vi "Frame Configuration Page.vi"(8 "error in (no error)":errorcluster, 11 "Node Ptr":T2 format="%.0x") -> (0 "error out":errorcluster)   [LabVIEW 2021, in "LIN Frame Protection Addon System Explorer.lvlib"]
uses:
  LIN Frame Protection Addon System Explorer.lvlib
  <vilib>/NI VeriStand/Custom Device API/Custom Device Item Ref.ctl
  Shared/Types/Protection Type.ctl
  <vilib>/NI VeriStand/Custom Device API/Custom Device API.lvlib
  Shared/LIN Frame Protection Addon Shared.lvlib
panel:
  out "Delays (s)":string
  in  "Protection Type":T1
  out "Frame ID":u32 format="%.0x"
  in  "Max Count":dbl=4.0
  out "Rolling Counter Channel":string
  out "CRC Channel":string
  in  "SHDocVw.IWebBrowser":refnum<k7>(container)
  in  "Value":dbl
  in  "Monitored Channels":i32(listbox)
  in  "Header":cluster{"Section Name":string}={"Section Name"="Custom Device Item Settings"}
  in  "Description":string
  in  "Name":string
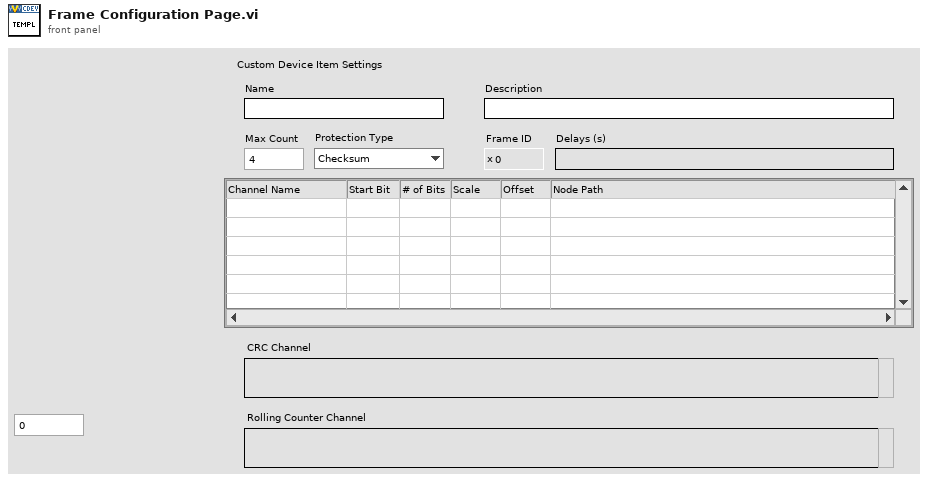
[diagram p1: front panel]
types:
  T1 = typedef "LIN Frame Protection Addon Shared.lvlib/Protection Type.ctl" = enum16{"Checksum", "CRC", "None (Counter Only)"}
  T2 = typedef "Custom Device API.lvlib/Custom Device Item Ref.ctl" = u64
  T3 = typedef "Custom Device API.lvlib/Custom Device Item Info.ctl" = cluster{"Name":string, "Is Channel":bool, "GUID":string, "Is Waveform":bool}
  T4 = typedef "LIN Frame Protection Addon Shared.lvlib/FrameConfiguration.ctl" = cluster{"Input Channels":T5[], "Schedule_SumOfDelays":cluster{"Index":i32, "Delays":dbl[]}, "Rolling Counter Count":dbl, "PCL Count":u64, "Max Count":dbl, "Frame ID":u32, "Rolling Counter":T5, "CRC":T5, "Frame Name":string, "Cluster":string, "Database":string, "Protection Type":T1}
  T5 = typedef "LIN Frame Protection Addon Shared.lvlib/InputChannelConfiguration.ctl" = cluster{"Start Bit":i32, "Name":string, "Node Path":string, "Number of bits":i32, "Scale":dbl, "Offset":dbl, "Data Type":u32}
  T6 = typedef "Custom Device API.lvlib/Custom Device Commands.ctl" = enum16{"Default", "Item renamed", "Shutdown", "Dynamic button pressed"}
  T7 = typedef "LVPoint32TypeDef.ctl" = cluster{"Horizontal":i32, "Vertical":i32}
  T8 = typedef "LVRowAndColumnTypeDef.ctl" = cluster{"Row":i32, "Column":i32}
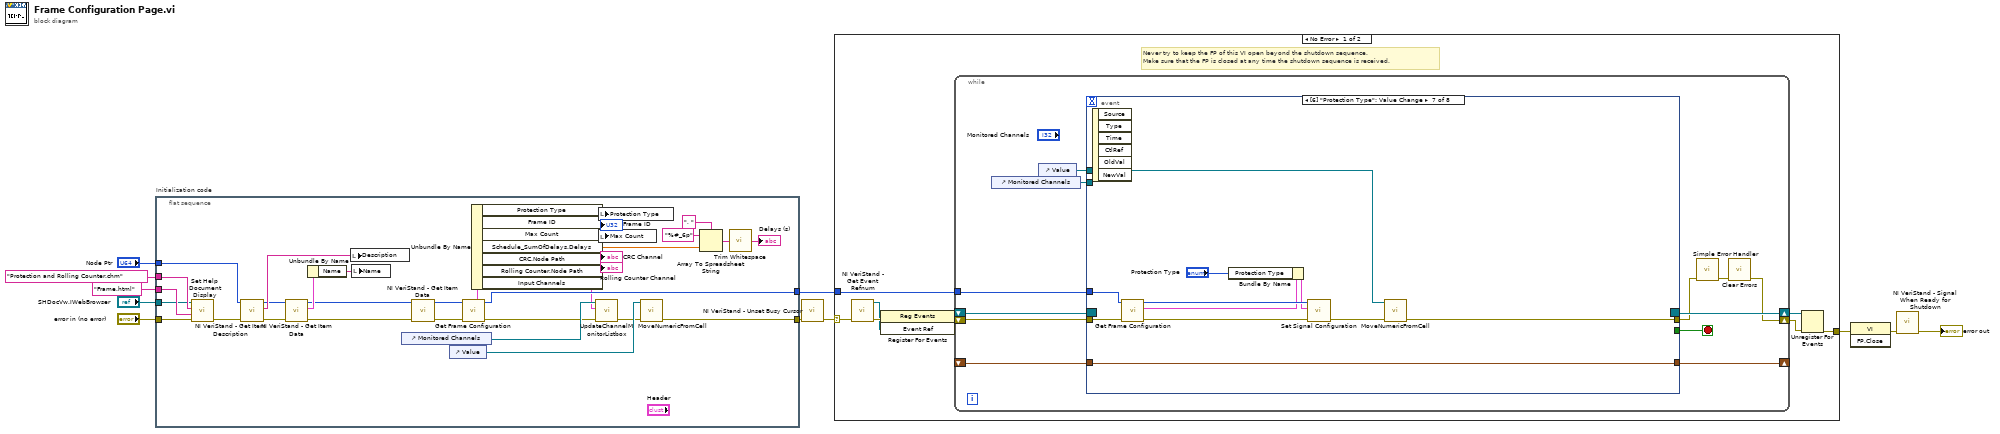
[diagram p0: block diagram]
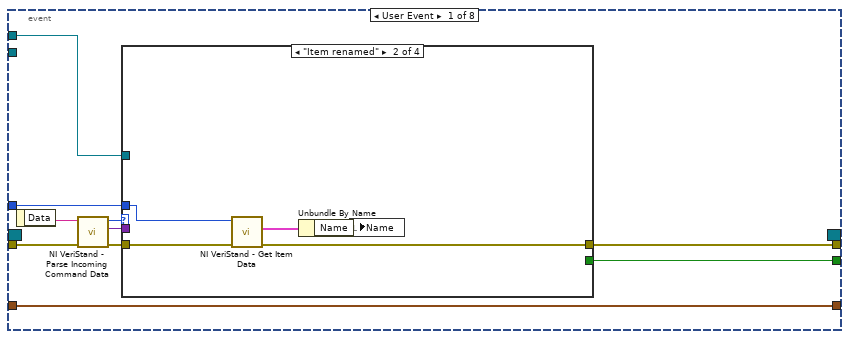
[diagram p2: hidden frame]
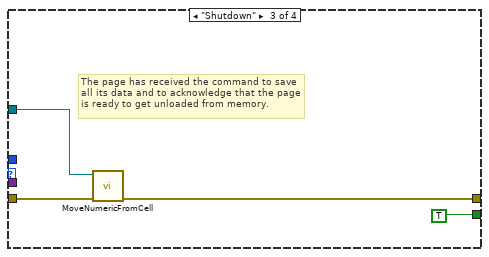
[diagram p4: hidden frame]
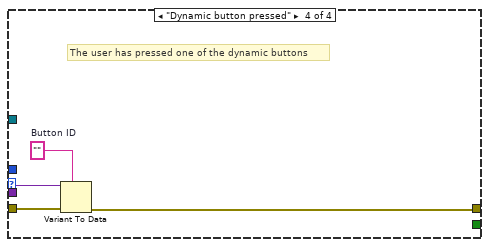
[diagram p5: hidden frame]
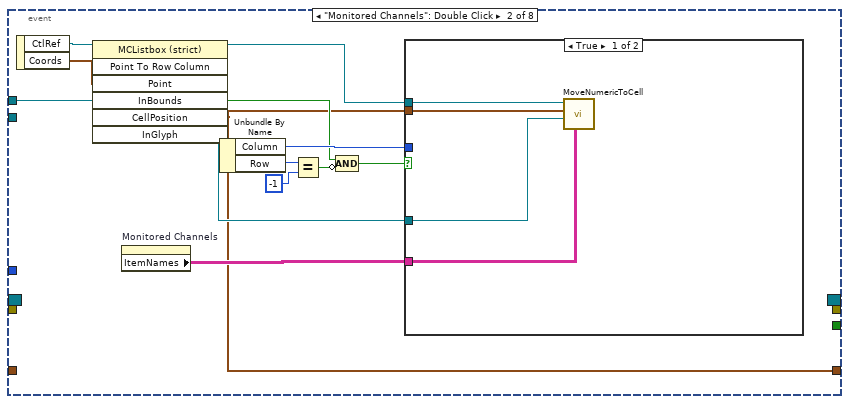
[diagram p6: hidden frame]
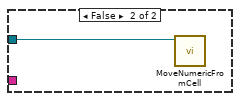
[diagram p7: hidden frame]
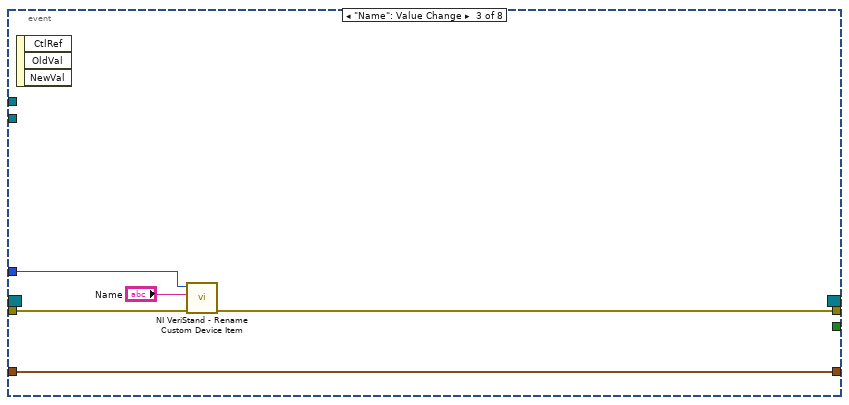
[diagram p8: hidden frame]
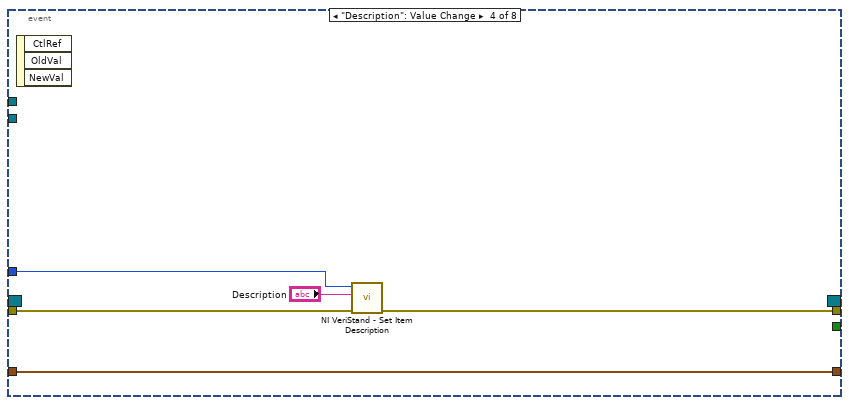
[diagram p9: hidden frame]
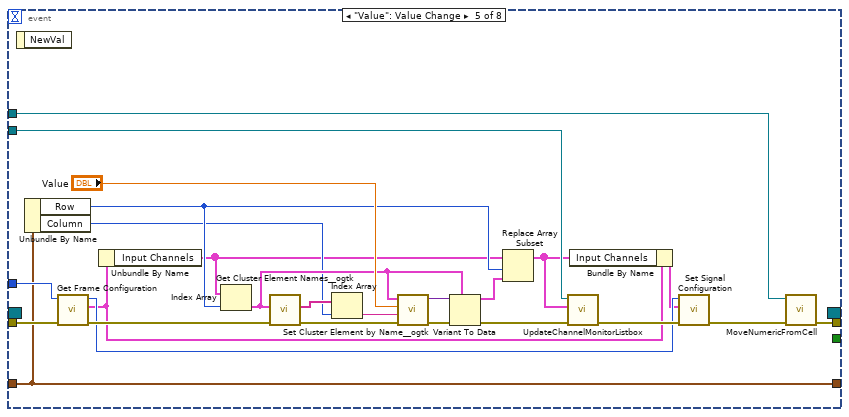
[diagram p10: hidden frame]
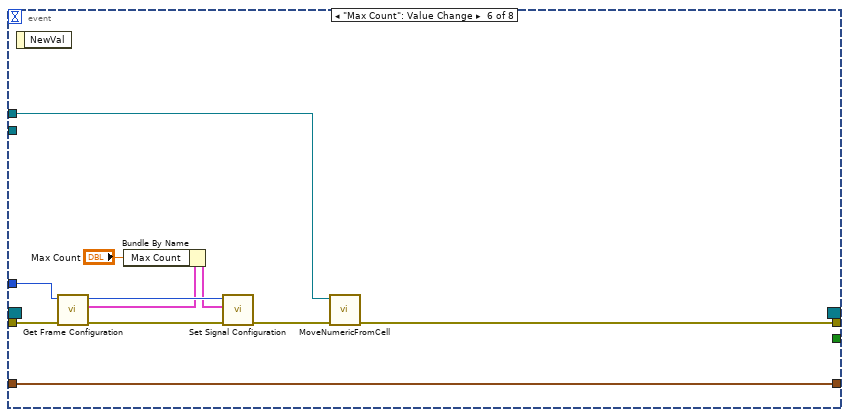
[diagram p11: hidden frame]
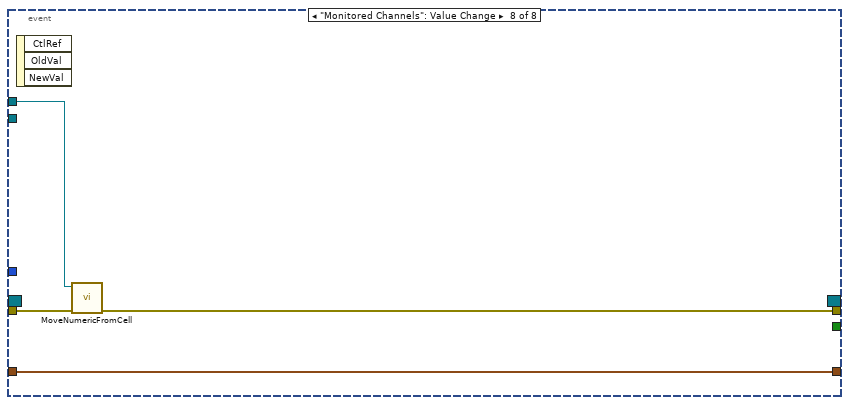
[diagram p12: hidden frame]
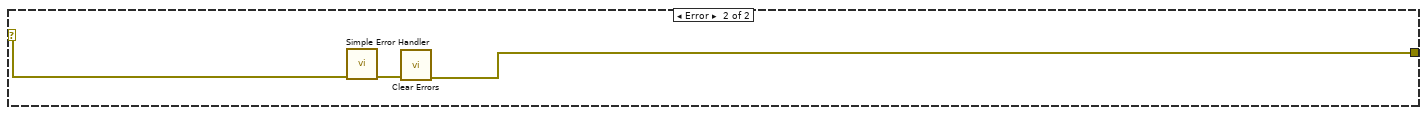
[diagram p13: hidden frame]
diagram:
  n1 = flat-sequence "Initialization code" {
    tunnel: "error in (no error)" -> [w35]
    tunnel: "Node Ptr" -> [w23]
    tunnel: [w32] -> w9
    tunnel: [w40] -> w7
    tunnel: "Protection and Rolling Counter.chm" ("Main CHM File") -> [w44]
    tunnel: "Frame.html" ("HTML File") -> [w43]
    tunnel: "SHDocVw.IWebBrowser" -> [w42]
    frame #0 {
      n2 = call "Set Help Document Display.vi"("error in (no error)"=w35, "HTML File"=w43, "Main CHM File"=w44, "SHDocVw.IWebBrowser2"=w42) -> ("error out"=w25:errorcluster)  [unwired: 7 in]
      n3 = call <vilib>:"NI VeriStand - Get Item Description.vi"("error in (no error)"=w25, "Item Ref in"=w23) -> ("error out"=w28:errorcluster, "Description"=w27:string, "Item Ref out"=w26:T2)  [unwired: 7 out]
      n4 = call <vilib>:"NI VeriStand - Get Item Data.vi"("error in (no error)"=w28, "Item Ref in"=w26) -> ("error out"=w24:errorcluster, "Item Info"=w29:T3, "Item Ref out"=w22:T2)  [unwired: 7 out]
      n5 = Unbundle By Name(w29) -> ("Name"=w30:string)
      n6 = local write "Description"(w27) -> ()
      n7 = local write "Name"(w30) -> ()
      n8 = control-ref of="Monitored Channels"() -> (w37:refnum<vi>)
      n9 = call <vilib>:"NI VeriStand - Get Item Data.vi"("error in (no error)"=w24, "Item Ref in"=w22) -> ("error out"=w39:errorcluster, "Item Ref out"=w41:T2)  [unwired: 8 out]
      n10 = control-ref of="Value"() -> (w34:refnum<vi>)
      n11 = call "Get Frame Configuration.vi"("error in"=w39, "Parent Ref"=w41) -> ("error out"=w36:errorcluster, "Selected Channels"=w38:T4, "Parent Ref Out"=w40:T2)  [unwired: 7 in]
      n12 = Unbundle By Name(w38) -> ("Protection Type"=w17:T1, "Frame ID"=→"Frame ID":u32, "Max Count"=w19:dbl, "Schedule_SumOfDelays.Delays"=w16:dbl[], "CRC.Node Path"=→"CRC Channel":string, "Rolling Counter.Node Path"=→"Rolling Counter Channel":string, "Input Channels"=w31:T5[])
      n13 = call "UpdateChannelMonitorListbox.vi"("error in (no error)"=w36, "Monitored Channels"=w31, "Listbox"=w37) -> ("error out"=w33:errorcluster)  [unwired: 8 in]
      n14 = local write "Protection Type"(w17) -> ()
      n15 = local write "Max Count"(w19) -> ()
      n16 = call "MoveNumericFromCell.vi"("error in (no error)"=w33, "Digital in"=w34) -> ("error out"=w32:errorcluster)  [unwired: 9 in]
      n17 = Array To Spreadsheet String(delimiter (Tab)=", ", array=w16, 3:"%#_6p" ("format string")) -> (spreadsheet string=w15:string)
      n18 = call <vilib>:"Trim Whitespace.vi"("string"=w15) -> ("trimmed string"=→"Delays (s)":string)  [unwired: 1 in]
    }
  }
  n19 = call <vilib>:"NI VeriStand - Unset Busy Cursor.vi"("error in (no error)"=w9) -> ("error out"=w8:errorcluster)  [unwired: 10 out]
  n20 = case shown="No Error" w8 {
    selector: w8 -> [w45 w170]
    tunnel: [w50 w168] -> w11
    tunnel: w7 -> [w46 _]
    frame No Error {
      # "Never try to keep the FP of this VI open beyond the shutdown sequence.\nMake sure that the FP is closed at any time the shutdown sequence is received."
      n21 = call <vilib>:"NI VeriStand - Get Event Refnum.vi"("error in (no error)"=w45) -> ("error out"=w53:errorcluster, "Event Ref"=w49:refnum<user-event>)  [unwired: 9 out]
      n22 = register-events(error in=w53, w49) -> (reference out=w47:refnum<event-registration>, error out=w48:errorcluster)  [unwired: 1 in]
      n23 = while {
        tunnel: w46 -> [w61]
        shift-right: [w58] -> w51
        shift-left: w48 -> [w64]
        shift-right: [w65] -> w52
        shift-left: w47 -> [w63]
        shift-right: [w56] -> _
        shift-left: _ -> [w55]
        stop <- w62 stop-if-true
        n24 = control-ref of="Monitored Channels"() -> (w54:refnum<vi>)
        n25 = control-ref of="Value"() -> (w57:refnum<vi>)
        n26 = event shown="[6] \"Protection Type\": Value Change" {
          selector: w63 -> [_ _ _ _ _ _ _ _]
          dyn-events: [_ _ _ _ _ _ _ _] -> w65
          timeout: _ -> [_ _ _ _ _ _ _ _]
          tunnel: w64 -> [w75 _ w109 w114 w139 w150 w161 w165]
          tunnel: [w71 _ _ _ _ _ _ _] -> w62
          tunnel: [w70 _ w107 w113 w123 w147 w158 w164] -> w60
          tunnel: w61 -> [w69 _ w108 w112 w140 w151 w162 _]
          tunnel: w57 -> [w66 w97 _ _ w141 w152 w163 w166]
          tunnel: [w67 w90 w111 w116 w135 w148 w159 w167] -> w56
          tunnel: w55 -> [w67 _ w111 w116 w135 w148 w159 w167]
          tunnel: w54 -> [_ _ _ _ w138 _ _ _]
          event User Event {
            n27 = event-data() -> ("Data"=w74:string)  [unwired: 1 out]
            n28 = call <vilib>:"NI VeriStand - Parse Incoming Command Data.vi"("error in (no error)"=w75, "Incoming data"=w74) -> ("error out"=w73:errorcluster, "Outgoing data"=w68:variant, "Action"=w72:T6)  [unwired: 7 out]
            n29 = case shown="\"Item renamed\"" w72 {
              tunnel: w73 -> [w76 w79 w83 w89]
              tunnel: [_ _ TRUE _] -> w71
              tunnel: [w76 w78 w82 w86] -> w70
              tunnel: w69 -> [_ w77 _ _]
              tunnel: w68 -> [_ _ _ w88]
              tunnel: w66 -> [_ _ w84 _]
              frame "Default", Default {
              }
              frame "Item renamed" {
                n30 = call <vilib>:"NI VeriStand - Get Item Data.vi"("error in (no error)"=w79, "Item Ref in"=w77) -> ("error out"=w78:errorcluster, "Item Info"=w80:T3)  [unwired: 8 out]
                n31 = Unbundle By Name(w80) -> ("Name"=w81:string)
                n32 = local write "Name"(w81) -> ()
              }
              frame "Shutdown" {
                # "The page has received the command to save all its data and to acknowledge that the page is ready to get unloaded from memory."
                n33 = call "MoveNumericFromCell.vi"("error in (no error)"=w83, "Digital in"=w84) -> ("error out"=w82:errorcluster)  [unwired: 9 in]
              }
              frame "Dynamic button pressed" {
                w87 = ""  # Button ID
                # "The user has pressed one of the dynamic buttons"
                n34 = Variant To Data(error in=w89, type=w87, Variant=w88) -> (error out=w86:errorcluster)  [unwired: 1 out]
              }
            }
          }
          event "Monitored Channels": Double Click {
            n35 = event-data() -> ("CtlRef"=w100:refnum<vi>, "Coords"=w99:T7)  [unwired: 1 out]
            n36 = invoke class="MCListbox (strict)" method="Point To Row Column"(reference=w100, "Point"=w99) -> (reference out=w98:refnum<vi>, "InBounds"=w94:bool, "CellPosition"=w90:T8)  [unwired: 5 in, 4 out]
            n37 = property on="Monitored Channels" class="MCListbox (strict)"() -> ("ItemNames"=w91:string[][])  [unwired: 2 in, 2 out]
            n38 = Unbundle By Name(w90) -> ("Column"=w101:i32, "Row"=w95:i32)
            n39 = Equal?(x=w95, y=-1) -> (x = y?=w93:bool)
            n40 = Compound Arithmetic op=AND(w94, invert w93) -> (w92:bool)
            n41 = case shown="True" w92 {
              tunnel: w101 -> [_ _]
              tunnel: w98 -> [w105 _]
              tunnel: w90 -> [w104 _]
              tunnel: w97 -> [w103 w106]
              tunnel: w91 -> [w102 _]
              frame True {
                n42 = call "MoveNumericToCell.vi"("Data"=w102, "Numeric"=w103, "Cell Position"=w104, "Listbox"=w105) -> ()  [unwired: 7 in, 1 out]
              }
              frame False {
                n43 = call "MoveNumericFromCell.vi"("Digital in"=w106) -> ()  [unwired: 10 in, 1 out]
              }
            }
          }
          event "Name": Value Change {
            n44 = event-data() -> ()  [unwired: 4 out]
            n45 = call <vilib>:"NI VeriStand - Rename Custom Device Item.vi"("error in (no error)"=w109, "New Name"="Name", "Item Ref in"=w108) -> ("error out"=w107:errorcluster)  [unwired: 1 in, 7 out]
          }
          event "Description": Value Change {
            n46 = event-data() -> ()  [unwired: 4 out]
            n47 = call <vilib>:"NI VeriStand - Set Item Description.vi"("error in (no error)"=w114, "Description"="Description", "Item Ref in"=w112) -> ("error out"=w113:errorcluster)  [unwired: 8 out]
          }
          event "Value": Value Change {
            n48 = event-data() -> ()  [unwired: 2 out]
            n49 = Unbundle By Name(w135) -> ("Row"=w124:i32, "Column"=w122:i32)
            n50 = call "Get Frame Configuration.vi"("error in"=w139, "Parent Ref"=w140) -> ("error out"=w128:errorcluster, "Selected Channels"=w119:T4, "Parent Ref Out"=w121:T2)  [unwired: 7 in]
            n51 = Unbundle By Name(w119) -> ("Input Channels"=w120:T5[])
            n52 = Index Array(array=w120, index=w124) -> (element=w126:T5)
            n53 = call <userlib>:"Get Cluster Element Names__ogtk.vi"("error in (no error)"=w128, "Cluster"=w126) -> ("error out"=w129:errorcluster, "Element Names"=w134:string[])  [unwired: 8 in]
            n54 = Index Array(array=w134, index=w122) -> (element=w133:string)
            n55 = call <userlib>:"Set Cluster Element by Name__ogtk.vi"("error in (no error)"=w129, "Element Name (\"\": New Element Data Name)"=w133, "New Element Value"="Value", "Cluster"=w126) -> ("error out"=w130:errorcluster, "VCluster out"=w131:variant)  [unwired: 5 in, 1 out]
            n56 = Variant To Data(error in=w130, type=w126, Variant=w131) -> (data=w125:T5, error out=w127:errorcluster)
            n57 = Replace Array Subset(array=w120, new element=w125, index=w124) -> (w118:T5[])
            n58 = call "UpdateChannelMonitorListbox.vi"("error in (no error)"=w127, "Monitored Channels"=w118, "Listbox"=w138) -> ("error out"=w137:errorcluster)  [unwired: 8 in]
            n59 = Bundle By Name(cluster=w119, "Input Channels"=w118) -> (w117:T4)
            n60 = call "Set Signal Configuration.vi"("error in"=w137, "Selected Channels"=w117, "Parent Ref"=w121) -> ("error out"=w136:errorcluster)  [unwired: 7 in, 1 out]
            n61 = call "MoveNumericFromCell.vi"("error in (no error)"=w136, "Digital in"=w141) -> ("error out"=w123:errorcluster)  [unwired: 9 in]
          }
          event "Max Count": Value Change {
            n62 = event-data() -> ()  [unwired: 2 out]
            n63 = call "Get Frame Configuration.vi"("error in"=w150, "Parent Ref"=w151) -> ("error out"=w143:errorcluster, "Selected Channels"=w145:T4, "Parent Ref Out"=w146:T2)  [unwired: 7 in]
            n64 = Bundle By Name(cluster=w145, "Max Count"="Max Count") -> (w144:T4)
            n65 = call "Set Signal Configuration.vi"("error in"=w143, "Selected Channels"=w144, "Parent Ref"=w146) -> ("error out"=w149:errorcluster)  [unwired: 7 in, 1 out]
            n66 = call "MoveNumericFromCell.vi"("error in (no error)"=w149, "Digital in"=w152) -> ("error out"=w147:errorcluster)  [unwired: 9 in]
          }
          event Value Change {
            n67 = event-data() -> ()  [unwired: 7 out]
            n68 = call "Get Frame Configuration.vi"("error in"=w161, "Parent Ref"=w162) -> ("error out"=w154:errorcluster, "Selected Channels"=w156:T4, "Parent Ref Out"=w157:T2)  [unwired: 7 in]
            n69 = Bundle By Name(cluster=w156, "Protection Type"="Protection Type") -> (w155:T4)
            n70 = call "Set Signal Configuration.vi"("error in"=w154, "Selected Channels"=w155, "Parent Ref"=w157) -> ("error out"=w160:errorcluster)  [unwired: 7 in, 1 out]
            n71 = call "MoveNumericFromCell.vi"("error in (no error)"=w160, "Digital in"=w163) -> ("error out"=w158:errorcluster)  [unwired: 9 in]
          }
          event "Monitored Channels": Value Change {
            n72 = event-data() -> ()  [unwired: 4 out]
            n73 = call "MoveNumericFromCell.vi"("error in (no error)"=w165, "Digital in"=w166) -> ("error out"=w164:errorcluster)  [unwired: 9 in]
          }
        }
        n74 = call <vilib>:"Simple Error Handler.vi"("error in (no error)"=w60) -> ("error out"=w59:errorcluster)  [unwired: 1 in, 7 out]
        n75 = call <vilib>:"Clear Errors.vi"("error in (no error)"=w59) -> ("error out"=w58:errorcluster)  [unwired: 1 in, 5 out]
      }
      n76 = Unregister For Events(event registration refnum=w52, error in=w51) -> (error out=w50:errorcluster)
    }
    frame Error {
      n77 = call <vilib>:"Simple Error Handler.vi"("error in (no error)"=w170) -> ("error out"=w169:errorcluster)  [unwired: 1 in, 7 out]
      n78 = call <vilib>:"Clear Errors.vi"("error in (no error)"=w169) -> ("error out"=w168:errorcluster)  [unwired: 1 in, 5 out]
    }
  }
  n79 = invoke class="VI" method="FP.Close"(error in=w11) -> (error out=w10:errorcluster)  [unwired: 2 in, 2 out]
  n80 = call <vilib>:"NI VeriStand - Signal When Ready for Shutdown.vi"("error in (no error)"=w10) -> ("error out"=→"error out":errorcluster)  [unwired: 10 out]
